vi "Resource Editor.vi"(7 "Load from Initial Path (F)":bool, 10 "Initial Resources":T1[](array[typedef]), 11 "Path":path) -> (2 "Final Resources":T1[](array[typedef]))   [LabVIEW 2026, in "VILab.lvlib"]
doc: "Edits several types of LabVIEW files at a low level, including VI's.\n\nCan also be used as a dialog subVI for editing resource clusters."
uses:
  VILab.lvlib
  CTLs/Resource.ctl
  CTLs/Resource Editor State Data.ctl
  <userlib>/_MGI/Application Control/MGI Gray if/MGI Gray if False.vi
  <vilib>/Utility/error.llb/Three Button Dialog (string).vi
  <vilib>/ErrorRing/Error Ring.xnode
  SubVIs/FaKI State Machine/FaKI State Machine.lvlib
panel:
  in  "Delete":bool
  in  "Add":bool
  in  "Name":string
  in  "Type":string
  in  "ID":i32
  in  "Export":bool
  in  "Import":bool
  in  "Paste":bool
  in  "Copy":bool
  in  "XML":bool
  in  "Fix MD5":bool
  in  "File type":string
  in  "Data":string
  in  "Hex view":bool
  in  "Save":bool
  in  "Load":bool
  in  "Resources":i32(listbox)=-1
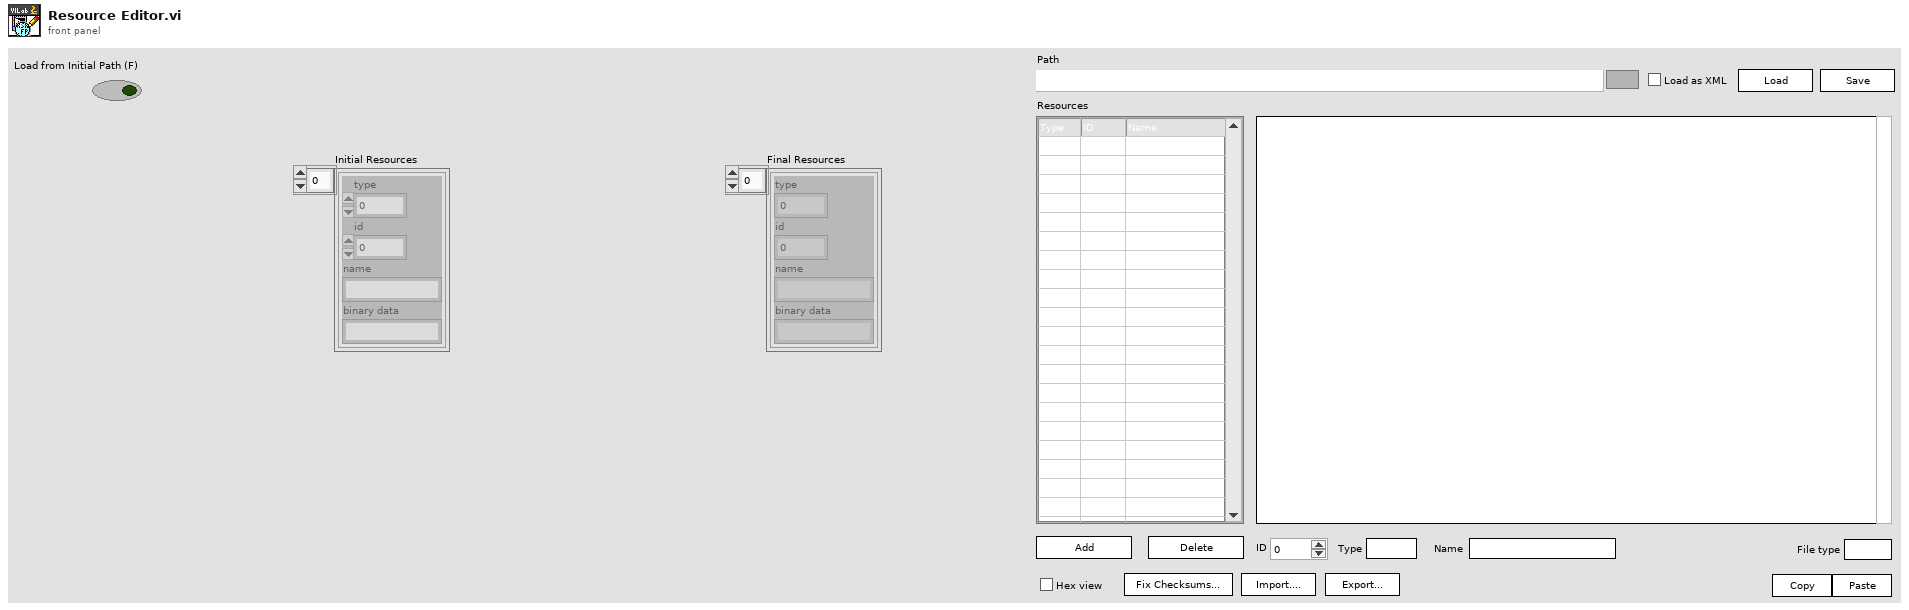
[diagram p1: front panel]
types:
  T1 = typedef "VILab.lvlib/Resource.ctl" = cluster{"type":u32, "id":i32, "name":string, "binary data":string}
  T2 = typedef "VILab.lvlib/Resource Editor State Data.ctl" = cluster{"Core":cluster{"Current VI Reference":refnum<vi>, "Close Panel on Exit?":bool}, "Path":path, "File Type":string, "Active Index":i32, "Active Resource":T1, "All Resources":T1[]}
  T3 = cluster{"format string":string, "Variant":variant}
  T4 = enum32{"Invalid", "Standard", "Closed", "Hidden", "Minimized", "Maximized"}
  T5 = enum32{"invalid app kind", "Development System", "Run Time System", "Student Edition", "Embedded LabVIEW", "Evaluation", "Custom"}
  T6 = enum16{"open", "replace", "create", "open or create", "replace or create", "replace or create with confirmation"}
  T7 = enum16{"Left Button", "Center Button", "Right Button", "Window Close"}
  T8 = enum8{"Enabled", "Disabled", "Disabled and Grayed Out"}
  T9 = typedef "VILab.lvlib/Terminal Counts.ctl" = cluster{"Numbers":u32, "Strings":u32, "Paths":u32}
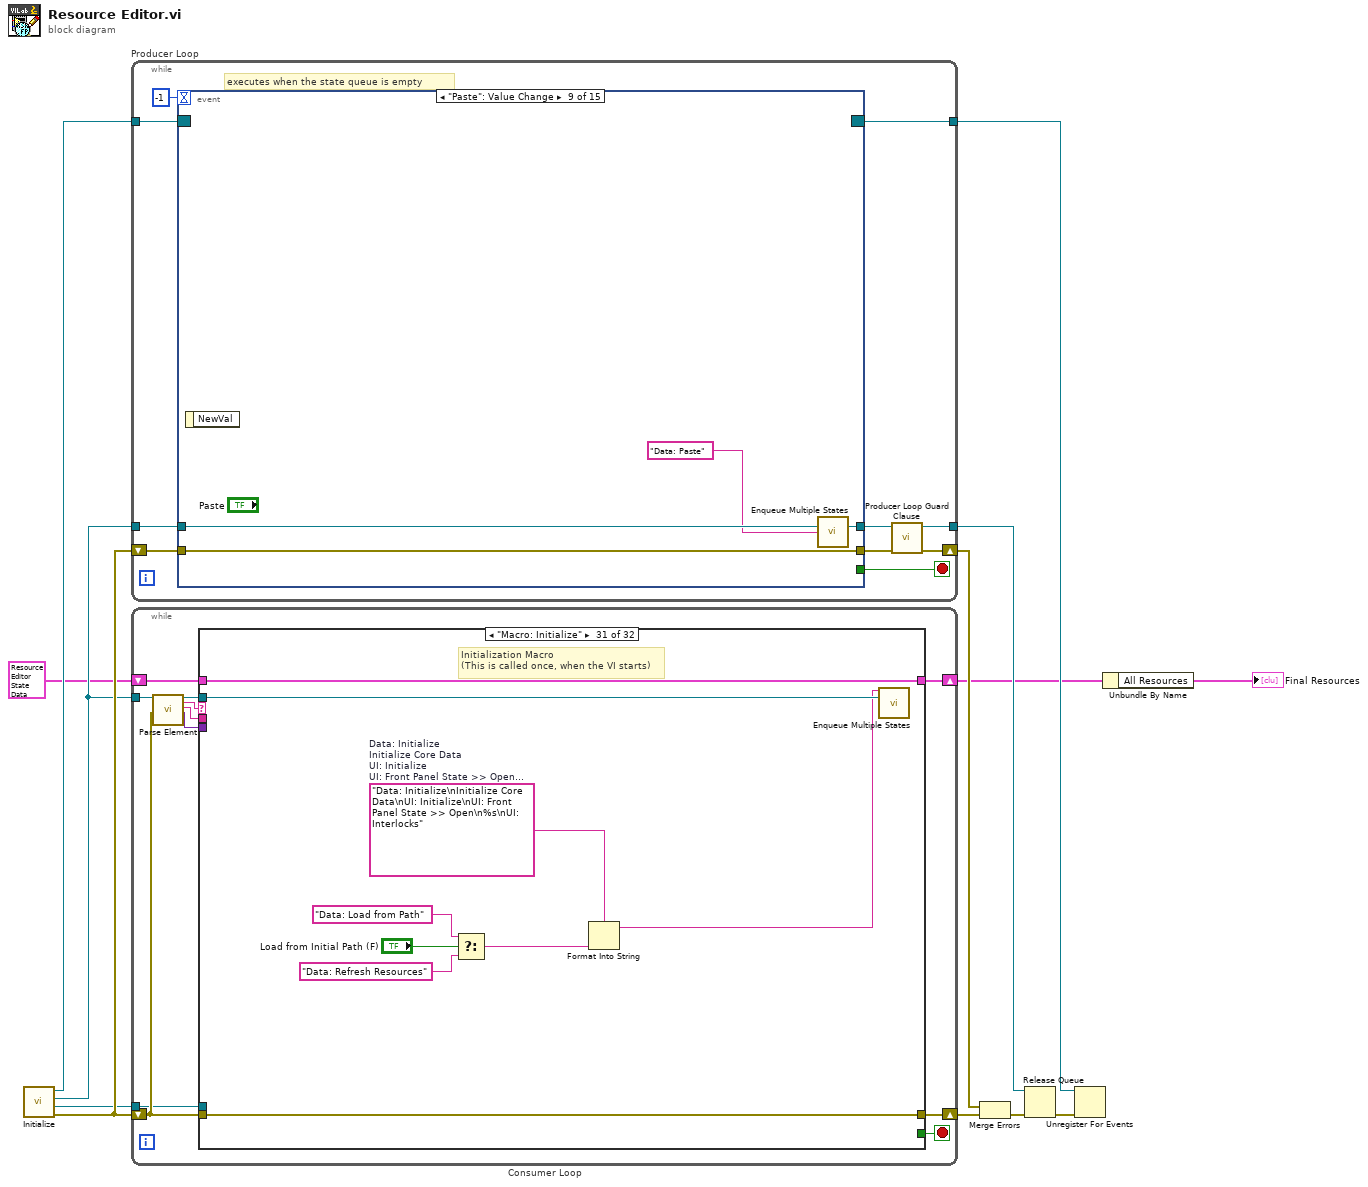
[diagram p0: block diagram]
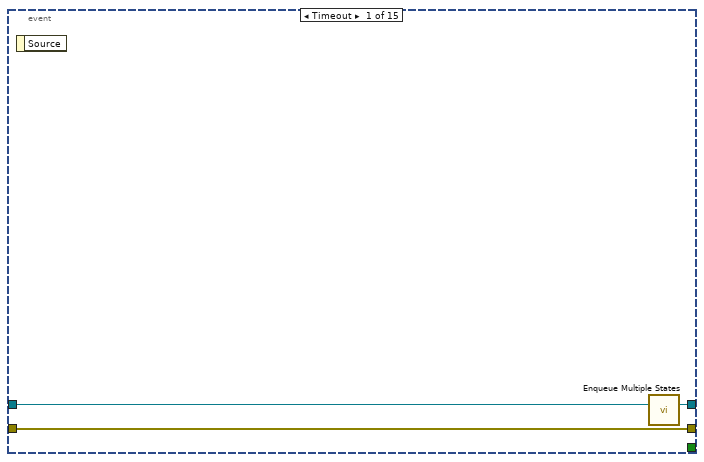
[diagram p2: hidden frame]
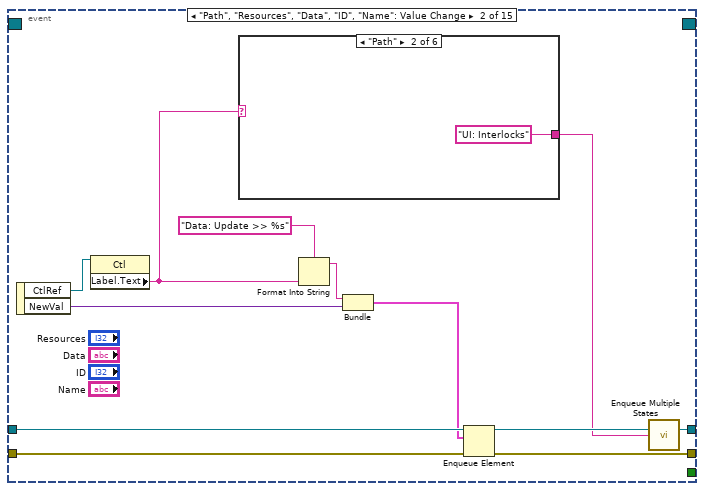
[diagram p3: hidden frame]
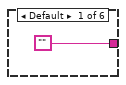
[diagram p4: hidden frame]
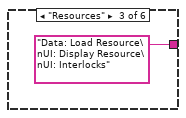
[diagram p5: hidden frame]
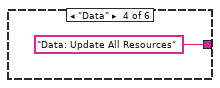
[diagram p6: hidden frame]
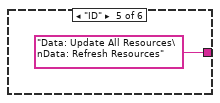
[diagram p7: hidden frame]
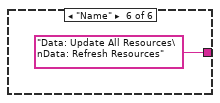
[diagram p8: hidden frame]
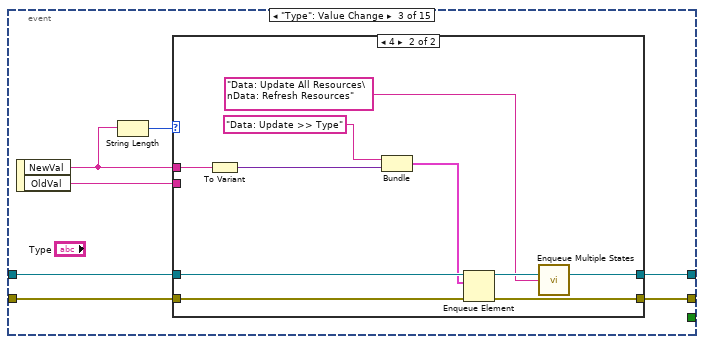
[diagram p9: hidden frame]
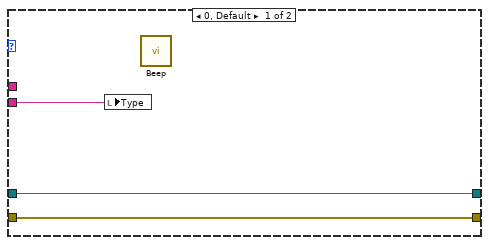
[diagram p10: hidden frame]
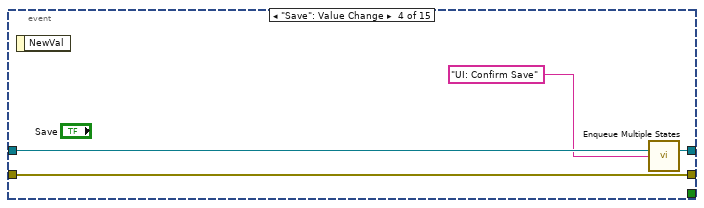
[diagram p11: hidden frame]
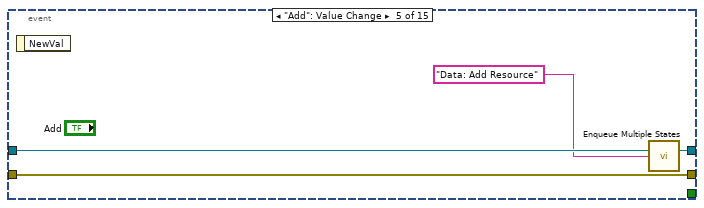
[diagram p12: hidden frame]
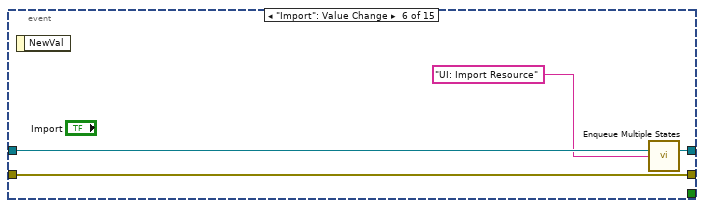
[diagram p13: hidden frame]
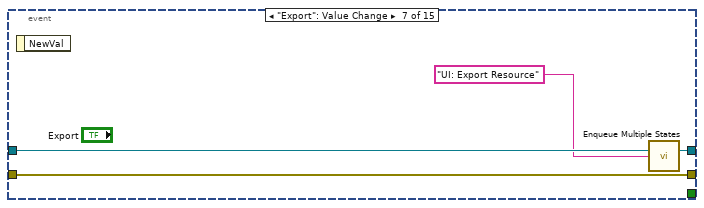
[diagram p14: hidden frame]
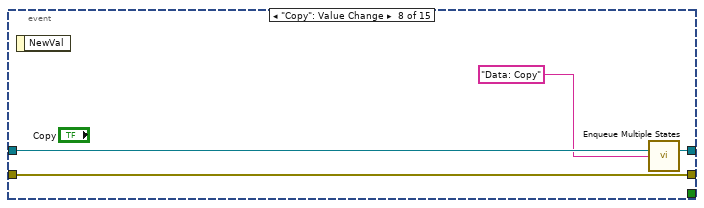
[diagram p15: hidden frame]
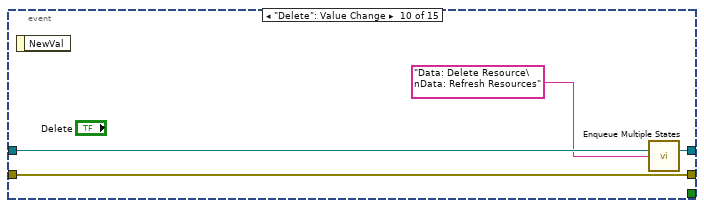
[diagram p16: hidden frame]
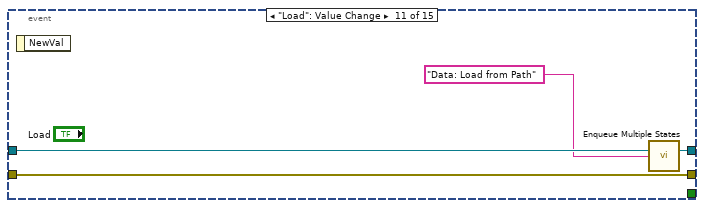
[diagram p17: hidden frame]
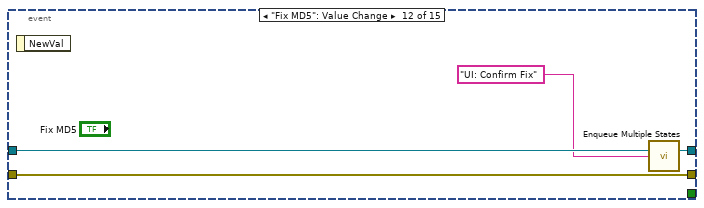
[diagram p18: hidden frame]
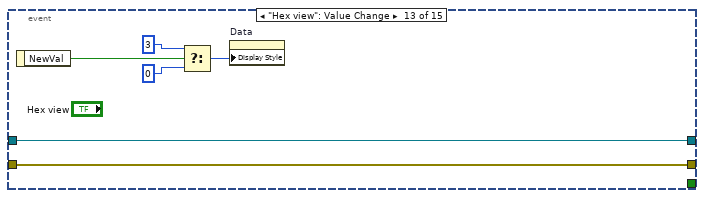
[diagram p19: hidden frame]
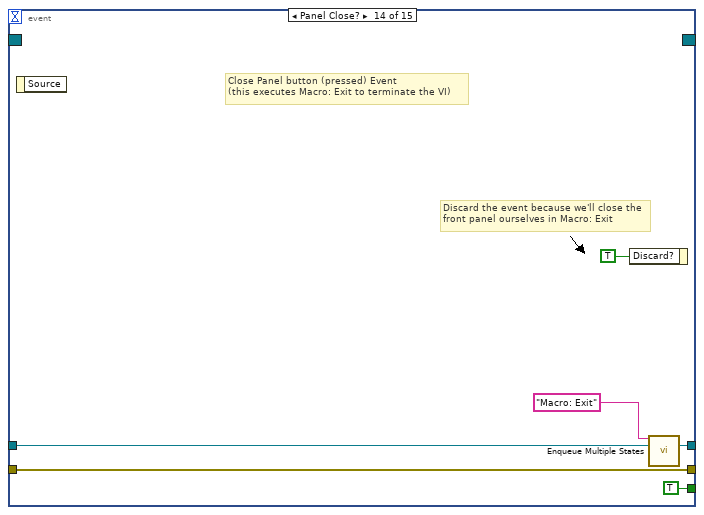
[diagram p20: hidden frame]
diagram:
  n1 = call "Initialize.vi"() -> ("error out"=w9:errorcluster, "Exit Event out"=w6:refnum<user-event>, "queue out"=w8:refnum<queue>, "Event Registration Refnum out"=w7:refnum<event-registration>)  [unwired: 8 in]
  n2 = while "Producer Loop" {
    shift-right: [w18] -> w12
    shift-left: w9 -> [w23]
    tunnel: w7 -> [w15]
    tunnel: w8 -> [w21]
    tunnel: [w16] -> w10
    tunnel: [w14] -> w4
    stop <- w20 stop-if-true
    # "executes when the state queue is empty"
    n3 = event shown="[8] \"Paste\": Value Change" {
      selector: w15 -> [_ _ _ _ _ _ _ _ _ _ _ _ _ _ _]
      dyn-events: [_ _ _ _ _ _ _ _ _ _ _ _ _ _ _] -> w14
      timeout: -1 ("Timeout") -> [_ _ _ _ _ _ _ _ _ _ _ _ _ _ _]
      tunnel: [w24 w36 w49 w67 w71 w75 w79 w83 w87 w91 w95 w99 w106 w112 w117] -> w19
      tunnel: w23 -> [w24 w37 w50 w67 w71 w75 w79 w83 w87 w91 w95 w99 w106 w112 w117]
      tunnel: w21 -> [w25 w35 w48 w66 w70 w74 w78 w82 w86 w90 w94 w98 w105 w109 w115]
      tunnel: [w26 w38 w51 w68 w72 w76 w80 w84 w88 w92 w96 w100 w105 w108 w114] -> w17
      tunnel: [_ _ _ _ _ _ _ _ _ _ _ _ _ TRUE TRUE] -> w20
      event Timeout {
        n4 = event-data() -> ()  [unwired: 1 in, 1 out]
        n5 = call "Enqueue Multiple States.vi"("queue in"=w25) -> ("queue out"=w26:refnum<queue>)  [unwired: 14 in]
      }
      event "Path", "Resources", "Data", "ID", "Name": Value Change {
        n6 = event-data() -> ("CtlRef"=w33:refnum<vi>, "NewVal"=w32:variant)  [unwired: 1 in]
        n7 = property class="Ctl"(reference=w33) -> ("Label.Text"=w29:string)  [unwired: 1 in, 2 out]
        n8 = case shown="\"Path\"" w29 {
          tunnel: ["" "UI: Interlocks" "Data: Load Resource\nUI: Display Resource\nUI: Interlocks" "Data: Update All Resources" "Data: Update All Resources\nData: Refresh Resources" "Data: Update All Resources\nData: Refresh Resources"] -> w27
          frame Default {
          }
          frame "Path" {
          }
          frame "Resources" {
          }
          frame "Data" {
          }
          frame "ID" {
          }
          frame "Name" {
          }
        }
        n9 = Format Into String(format string="Data: Update >> %s", w29) -> (resulting string=w30:string)  [unwired: 2 in, 1 out]
        n10 = Bundle(w30, "NewVal"=w32) -> (w28:cluster{string, "NewVal":variant})  [unwired: 1 in]
        n11 = Enqueue Element(queue=w35, element=w28, error in (no error)=w37) -> (queue out=w34:refnum<queue>, error out=w36:errorcluster)  [unwired: 1 in, 1 out]
        n12 = call "Enqueue Multiple States.vi"("queue in"=w34, "State(s) at Back"=w27) -> ("queue out"=w38:refnum<queue>)  [unwired: 13 in]
      }
      event "Type": Value Change {
        n13 = event-data() -> ("NewVal"=w47:string, "OldVal"=w45:string)  [unwired: 1 in]
        n14 = String Length(string=w47) -> (length=w46:i32)
        n15 = case shown="4" w46 {
          tunnel: [w54 w64] -> w51
          tunnel: w50 -> [w53 w63]
          tunnel: [w53 w62] -> w49
          tunnel: w48 -> [w54 w61]
          tunnel: w47 -> [_ w56]
          tunnel: w45 -> [w52 _]
          frame 0, Default {
            n16 = local write "Type"(w52) -> ()
            n17 = call <vilib>:"Beep.vi"() -> ()  [unwired: 12 in]
          }
          frame 4 {
            n18 = To Variant(anything=w56) -> (Variant=w55:variant)
            n19 = Bundle("format string"="Data: Update >> Type", "Variant"=w55) -> (w58:T3)  [unwired: 1 in]
            n20 = Enqueue Element(queue=w61, element=w58, error in (no error)=w63) -> (queue out=w60:refnum<queue>, error out=w62:errorcluster)  [unwired: 1 in, 1 out]
            n21 = call "Enqueue Multiple States.vi"("queue in"=w60, "State(s) at Back"="Data: Update All Resources\nData: Refresh Resources") -> ("queue out"=w64:refnum<queue>)  [unwired: 13 in]
          }
        }
      }
      event "Save": Value Change {
        n22 = event-data() -> ()  [unwired: 1 in, 1 out]
        n23 = call "Enqueue Multiple States.vi"("queue in"=w66, "State(s) at Back"="UI: Confirm Save") -> ("queue out"=w68:refnum<queue>)  [unwired: 13 in]
      }
      event "Add": Value Change {
        n24 = event-data() -> ()  [unwired: 1 in, 1 out]
        n25 = call "Enqueue Multiple States.vi"("queue in"=w70, "State(s) at Back"="Data: Add Resource") -> ("queue out"=w72:refnum<queue>)  [unwired: 13 in]
      }
      event "Import": Value Change {
        n26 = event-data() -> ()  [unwired: 1 in, 1 out]
        n27 = call "Enqueue Multiple States.vi"("queue in"=w74, "State(s) at Back"="UI: Import Resource") -> ("queue out"=w76:refnum<queue>)  [unwired: 13 in]
      }
      event "Export": Value Change {
        n28 = event-data() -> ()  [unwired: 1 in, 1 out]
        n29 = call "Enqueue Multiple States.vi"("queue in"=w78, "State(s) at Back"="UI: Export Resource") -> ("queue out"=w80:refnum<queue>)  [unwired: 13 in]
      }
      event "Copy": Value Change {
        n30 = event-data() -> ()  [unwired: 1 in, 1 out]
        n31 = call "Enqueue Multiple States.vi"("queue in"=w82, "State(s) at Back"="Data: Copy") -> ("queue out"=w84:refnum<queue>)  [unwired: 13 in]
      }
      event "Paste": Value Change {
        n32 = event-data() -> ()  [unwired: 1 in, 1 out]
        n33 = call "Enqueue Multiple States.vi"("queue in"=w86, "State(s) at Back"="Data: Paste") -> ("queue out"=w88:refnum<queue>)  [unwired: 13 in]
      }
      event "Delete": Value Change {
        n34 = event-data() -> ()  [unwired: 1 in, 1 out]
        n35 = call "Enqueue Multiple States.vi"("queue in"=w90, "State(s) at Back"="Data: Delete Resource\nData: Refresh Resources") -> ("queue out"=w92:refnum<queue>)  [unwired: 13 in]
      }
      event "Load": Value Change {
        n36 = event-data() -> ()  [unwired: 1 in, 1 out]
        n37 = call "Enqueue Multiple States.vi"("queue in"=w94, "State(s) at Back"="Data: Load from Path") -> ("queue out"=w96:refnum<queue>)  [unwired: 13 in]
      }
      event "Fix MD5": Value Change {
        n38 = event-data() -> ()  [unwired: 1 in, 1 out]
        n39 = call "Enqueue Multiple States.vi"("queue in"=w98, "State(s) at Back"="UI: Confirm Fix") -> ("queue out"=w100:refnum<queue>)  [unwired: 13 in]
      }
      event "Hex view": Value Change {
        n40 = event-data() -> ("NewVal"=w101:bool)  [unwired: 1 in]
        n41 = Select(t=u32 3 ("Display Style"), s=w101, f=u32 0 ("Display Style")) -> (s? t:f=w104:u32)
        n42 = property on="Data" class="Str"("Display Style"=w104) -> ()  [unwired: 2 in, 2 out]
      }
      event Panel Close? {
        # "Discard the event because we'll close the front panel ourselves in Macro: Exit"
        # "Close Panel button (pressed) Event\n(this executes Macro: Exit to terminate the VI)"
        n43 = event-data() -> ()  [unwired: 1 in, 1 out]
        n44 = event-data("Discard?"=TRUE) -> ()  [unwired: 1 in, 1 out]
        n45 = call "Enqueue Multiple States.vi"("State(s) at Front"="Macro: Exit", "queue in"=w109) -> ("queue out"=w108:refnum<queue>)  [unwired: 13 in]
      }
      event User Event {
        # "\"Exit\" Dynamic Event registered\n(this executes Macro: Exit to terminate the VI)"
        n46 = event-data() -> ()  [unwired: 1 in, 5 out]
        n47 = call "Enqueue Multiple States.vi"("State(s) at Front"="Macro: Exit", "queue in"=w115) -> ("queue out"=w114:refnum<queue>)  [unwired: 13 in]
      }
    }
    n48 = call "Producer Loop Guard Clause.vi"("error in (no error)"=w19, "queue in"=w17) -> ("error out"=w18:errorcluster, "queue out"=w16:refnum<queue>)  [unwired: 8 in]
  }
  n49 = while "Consumer Loop" {
    shift-right: [w125] -> w2
    shift-left: T2 {"Core"={"Current VI Reference"=refnum, "Close Panel on Exit?"=FALSE}, "Path"=path "", "File Type"="", "Active Index"=0, "Active Resource"={"type"=0, "id"=0, "name"="", "binary data"=""}, "All Resources"=[]} ("Resource Editor State Data") -> [w124]
    shift-right: [w128] -> w13
    shift-left: w9 -> [w127]
    tunnel: w8 -> [w123]
    tunnel: w6 -> [w118]
    stop <- w126 stop-if-true
    n50 = call "Parse Element.vi"("queue in"=w123, "error in (no error)"=w127) -> ("queue out"=w122:refnum<queue>, "State"=w121:string, "Arg"=w120:string, "Data"=w119:variant)  [unwired: 14 in]
    n51 = case shown="\"Macro: Initialize\"" w121 {
      selector: w121 -> [_ w133 _ _ _ _ _ _ _ _ _ _ _ _ _ _ _ _ _ _ _ _ _ _ _ _ _ _ _ _ _ _]
      tunnel: w122 -> [w129 w132 w142 w158 _ w164 _ _ w243 _ _ _ _ _ w297 w327 _ _ _ _ w415 w419 w428 w431 w440 _ _ _ _ w586 w595 w602]
      tunnel: w120 -> [_ _ _ w154 _ _ _ w175 _ _ _ _ _ _ _ _ _ _ _ _ _ _ _ w432 w441 _ _ _ _ _ _ _]
      tunnel: w124 -> [w130 w135 w148 w159 w162 w165 w169 w176 w242 w255 w266 w272 w282 w288 w304 w330 w344 w355 w364 w396 w416 w420 w429 w433 w443 w518 w523 w535 w551 w587 w596 w606]
      tunnel: [w131 w140 w153 errorcluster {"status"=FALSE, "code"=0, "source"=""} ("error out") w163 w166 w170 w171 w232 w257 w267 w273 w283 w289 w298 w328 w342 w356 w365 w390 w418 w421 w430 w434 w444 w516 w529 w530 w552 w588 w597 w607] -> w128
      tunnel: w127 -> [w131 w139 w153 w157 w163 w166 w170 w174 w234 w257 w267 w273 w283 w289 w299 w329 w345 w356 w365 w397 w414 w421 w430 w435 w445 w522 w529 w532 w552 w588 w597 w607]
      tunnel: [_ _ _ _ TRUE _ _ _ _ _ _ _ _ _ _ _ _ _ _ _ _ _ _ _ _ _ _ _ _ _ _ _] -> w126
      tunnel: [w130 w135 w152 w159 w162 w165 w168 w172 w238 w255 w265 w271 w281 w287 w304 w330 w343 w354 w363 w395 w416 w420 w429 w433 w443 w518 w523 w535 w550 w587 w596 w606] -> w125
      tunnel: w119 -> [_ _ _ w155 _ _ _ w173 _ _ _ _ _ _ _ _ w341 _ _ w394 _ _ _ _ _ _ _ _ _ _ _ _]
      tunnel: w118 -> [_ _ _ _ _ _ _ _ _ _ _ _ _ _ _ _ _ _ _ _ w413 _ _ _ _ _ _ _ _ _ _ _]
      frame "---------- Core ----------" {
        # "Do not put any code in this frame.\n(it is a separator no-op)"
        n52 = call "Enqueue Multiple States.vi"("queue in"=w129) -> ()  [unwired: 14 in, 1 out]
      }
      frame Default {
        w137 = 42 items=["No error", "Argument error", "Memory is full", "Out of zone", "End of file", "File already open", "Generic file I/O error", "File not found", "File permission error", "Disk is full", "Duplicate path", "Too many files open", "System feature not enabled", "Resource file not found", "Cannot add resource", "Resource not found", "Image not found", "Image memory error", "Pen does not exist", "Config type invalid", "Config token not found", "Config parse error", "Config memory error", "Bad external code format", "Bad external code offset", "External code not present", "Null window", "Destroy window error", "Null menu", "Print aborted", "Bad print record", "Print driver error", "Windows error during printing", "Memory error during printing", "Print dialog error", "Generic print error", "Invalid device refnum", "Device not found", "Device parameter error", "Device unit error", "Cannot open device", "Device call aborted", "Generic error", "Cancelled by user", "Object ID too low", "Object ID too high", "Object not in heap", "Unknown heap", "Unknown object (invalid DefProc)", "Unknown object (DefProc not in table)", "Message out of range", "Invalid (null) method", "Unknown message", "Manager call not supported", "Bad address", "Network operation in progress", "Network operation timed out", "Connection is busy", "Network attribute not supported", "Network error", "Address in use", "System out of memory", "Connection aborted", "Connection refused", "Not connected", "Already connected", "Connection closed", "Initialization error (interapplication manager)", "Bad occurrence", "Wait on unbound occurrence handler", "Occurrence queue overflow", "Datalog type conflict", "Unused", "Unrecognized type (interapplication manager)", "Memory corrupt", "Failed to make temporary DLL", "Old CIN version", "Drag socket not found", "Failed to load drop-object", "Failed to register OLE object", "Failed to release OLE object", "Format specifier type mismatch", "Unknown format specifier", "Too few format specifiers", "Too many format specifiers", "Scan failed", "Newer CIN version", "Error converting to variant", "Runtime menu error", "Password tampered", "Variant attribute not found", "Incompatible variant data type", "Event data is not available", "Event Store is not present", "Occurrence is not found", "Event Queue is not created", "Event info is not available", "Refnum passed is NULL", "Error retrieving Class GUID", "Error retrieving CoClass GUID", "Error retrieving TypeLib GUID.", "Bad built application magic bytes.", "Specific driver is different from the specific driver associated with the Logical Name.", "There is no session opened to the class driver.", "Max Error", "MAX - Error with config objects", "MAX - Error loading configuration", "MAX - Group not supported"]
        # "Current State"
        # "Do not delete, rename, or modify this frame.\n(this is used to capture unhandled states and typos)"
        # "Handle mistyped state name (developer tool)"
        n53 = Format Into String(format string="Software Exception: Unhandled State \"%s\"." ("message"), error in=w139, w133) -> (resulting string=w136:string, error out=w141:errorcluster)  [unwired: 1 in]
        n54 = call <vilib>:"Error Cluster From Error Code.vi"("show call chain? (False)"=TRUE, "error in (no error)"=w141, "error message (\"\")"=w136, "error code (0)"=w137) -> ("error out"=w140:errorcluster)  [unwired: 5 in]
        n55 = call "Enqueue Multiple States.vi"("queue in"=w132) -> ()  [unwired: 14 in, 1 out]
      }
      frame "Initialize Core Data" {
        # "Do not delete, rename, or modify this frame.\n(this is used to determine panel behavior on exit)"
        # "originally closed?"
        # "exe?"
        # "If panel starts closed or is an EXE, then close it when we exit"
        n56 = property class="VI"() -> ("FP.State"=w145:T4)  [unwired: 2 in, 2 out]
        n57 = property class="App"() -> ("App.Kind"=w151:T5)  [unwired: 2 in, 2 out]
        n58 = control-ref of="Current VI Reference"() -> (w146:refnum<vi>)
        n59 = Equal?(x=w145, y=T4."Closed" ("Front Panel Window:State")) -> (x = y?=w143:bool)
        n60 = Equal?(x=w151, y=T5."Run Time System" ("Application:Kind")) -> (x = y?=w149:bool)
        n61 = Or(x=w143, y=w149) -> (x .or. y?=w147:bool)
        n62 = Bundle By Name(cluster=w148, "Core.Current VI Reference"=w146, "Core.Close Panel on Exit?"=w147) -> (w152:T2)
        n63 = call "Enqueue Multiple States.vi"("queue in"=w142) -> ()  [unwired: 14 in, 1 out]
      }
      frame "Error Handler" {
        # "Unhandled Error -- Display it"
        # "Handle any errors here.\nYou can also output any states to clean-up after errors occur"
        # "Clear error"
        n64 = call "Build Error Message.vi"("error in (no error)"=w157, "Data"=w155, "Arg"=w154) -> ("error out"=w156:errorcluster)  [unwired: 8 in]
        n65 = call <vilib>:"General Error Handler.vi"("error in (no error)"=w156) -> ()  [unwired: 10 in, 5 out]
        n66 = call "Enqueue Multiple States.vi"("queue in"=w158) -> ()  [unwired: 14 in, 1 out]
      }
      frame "Exit" {
        # "Do not put any code in this frame.\n(No errors that occur here will be handled.)"
      }
      frame "---------- Data ----------" {
        # "Do not put any code in this frame.\n(It is a separator no-op. You can make a copy of this frame to create a new Data frame)"
        n67 = call "Enqueue Multiple States.vi"("queue in"=w164) -> ()  [unwired: 14 in, 1 out]
      }
      frame "Data: Initialize" {
        # "Initialize the shift-register data, here."
        n68 = Bundle By Name(cluster=w169, "All Resources"="Initial Resources") -> (w168:T2)
      }
      frame "Data: Update" {
        n69 = case shown="\"Name\"" w175 {
          selector: w175 -> [w177 _ _ _ _ _ _]
          tunnel: w176 -> [w179 w190 w197 w204 w213 w220 w227]
          tunnel: w174 -> [_ w193 w200 w207 w216 w223 w230]
          tunnel: w173 -> [_ w191 w198 w205 w214 w221 w228]
          tunnel: [w179 w189 w196 w203 w212 w219 w226] -> w172
          tunnel: [w178 w187 w194 w201 w211 w218 w225] -> w171
          frame Default {
            n70 = xnode "Error Ring"("parameter 0"=w177) -> ("error out"=w178:errorcluster)
          }
          frame "Path" {
            n71 = Variant To Data(error in=w193, type=path "", Variant=w191) -> (data=w188:path, error out=w187:errorcluster)
            n72 = Bundle By Name(cluster=w190, "Path"=w188) -> (w189:T2)
          }
          frame "Resources" {
            n73 = Variant To Data(error in=w200, type=0, Variant=w198) -> (data=w195:i32, error out=w194:errorcluster)
            n74 = Bundle By Name(cluster=w197, "Active Index"=w195) -> (w196:T2)
          }
          frame "Data" {
            n75 = Variant To Data(error in=w207, type="", Variant=w205) -> (data=w202:string, error out=w201:errorcluster)
            n76 = Bundle By Name(cluster=w204, "Active Resource.binary data"=w202) -> (w203:T2)
          }
          frame "Type" {
            n77 = Variant To Data(error in=w216, type="", Variant=w214) -> (data=w209:string, error out=w211:errorcluster)
            n78 = Type Cast(type=u32 0, x=w209) -> (*(type *) &x=w208:u32)
            n79 = Bundle By Name(cluster=w213, "Active Resource.type"=w208) -> (w212:T2)
          }
          frame "ID" {
            n80 = Variant To Data(error in=w223, type=0, Variant=w221) -> (data=w217:i32, error out=w218:errorcluster)
            n81 = Bundle By Name(cluster=w220, "Active Resource.id"=w217) -> (w219:T2)
          }
          frame "Name" {
            n82 = Variant To Data(error in=w230, type="", Variant=w228) -> (data=w224:string, error out=w225:errorcluster)
            n83 = Bundle By Name(cluster=w227, "Active Resource.name"=w224) -> (w226:T2)
          }
        }
      }
      frame "Data: Load from Path" {
        n84 = case shown="True" "XML" {
          tunnel: "Path" -> [w245 w253]
          tunnel: [w245 w248] -> w239
          tunnel: w234 -> [w244 w247]
          tunnel: [w244 w246] -> w233
          frame False {
          }
          frame True {
            n85 = Open VI Reference(vi path=w253, error in (no error)=w247) -> (vi reference=w252:refnum<vi>, error out=w251:errorcluster)  [unwired: 4 in]
            n86 = call "Save VI with XML Heaps.vi"("error in (no error)"=w251, "VI Refnum In"=w252) -> ("error out"=w250:errorcluster, "VI Path out"=w248:path, "VI Refnum Out"=w249:refnum<vi>)  [unwired: 7 in]
            n87 = Close Reference(reference=w249, error in (no error)=w250) -> (error out=w246:errorcluster)
          }
        }
        n88 = property on="Resources" class="MCListbox (strict)"("Val(Sgnl)"=0 ("Value (Signaling)")) -> ()  [unwired: 2 in, 2 out]
        n89 = call "Load Resource File.vi"("error in (no error)"=w233, "Resource File"=w239) -> ("error out"=w232:errorcluster, "File Type"=w231:string, "Resources"=w237:T1[])  [unwired: 7 in]
        n90 = Bundle By Name(cluster=w242, "All Resources"=w237, "File Type"=w231) -> (w238:T2)
        n91 = local write "File type"(w231) -> ()
        n92 = call "Enqueue Multiple States.vi"("queue in"=w243, "State(s) at Back"="Data: Refresh Resources") -> ()  [unwired: 13 in, 1 out]
      }
      frame "Data: Refresh Resources" {
        n93 = Unbundle By Name(w255) -> ("All Resources"=w254:T1[])
        n94 = for {
          tunnel: [w264] -> w256 mode=indexing
          tunnel: w254 -> [w260] mode=indexing
          n95 = Unbundle By Name(w260) -> ("type"=w263:u32, "id"=w259:i32, "name"=w258:string)
          n96 = Type Cast(x=w263) -> (*(type *) &x=w261:string)  [unwired: 1 in]
          n97 = Number To Decimal String(number=w259) -> (decimal integer string=w262:string)  [unwired: 1 in]
          n98 = Build Array(w261, w262, w258) -> (w264:string[])
        }
        n99 = property on="Resources" class="MCListbox (strict)"("ItemNames"=w256) -> ()  [unwired: 2 in, 2 out]
      }
      frame "Data: Delete Resource" {
        n100 = in-place {
          n101 = in-place-cluster #1(w266) -> ("All Resources"=w270:T1[], "Active Index"=w268:i32)
          n102 = Delete From Array(array=w270, index=w268) -> (array with subset deleted=w269:T1[])  [unwired: 1 in, 1 out]
          n103 = in-place-cluster #1("All Resources"=w269, "Active Index"=w268) -> (w265:T2)
        }
      }
      frame "Data: Add Resource" {
        n104 = in-place {
          n105 = in-place-cluster #2(w272) -> ("All Resources"=w276:T1[], "Active Index"=w274:i32)
          n106 = property on="Resources" class="MCListbox (strict)"() -> ("ItemNames"=w280:string[][])  [unwired: 2 in, 2 out]
          n107 = Insert Into Array(array=w280, index (row)=w274, new element=string[] ["NewR", "0", ""]) -> (w279:string[][])  [unwired: 1 in]
          n108 = Insert Into Array(array=w276, index=w274, new element=T1 {"type"=1315272530, "id"=0, "name"="", "binary data"=""} ("element")) -> (w275:T1[])
          n109 = property on="Resources" class="MCListbox (strict)"("ItemNames"=w279, "Val(Sgnl)"=w274) -> ()  [unwired: 2 in, 2 out]
          n110 = in-place-cluster #2("All Resources"=w275, "Active Index"=w274) -> (w271:T2)
        }
      }
      frame "Data: Load Resource" {
        n111 = in-place {
          n112 = in-place-cluster #3(w282) -> ("All Resources"=w285:T1[], "Active Index"=w286:i32)  [unwired: 1 out]
          n113 = Index Array(array=w285, index=w286) -> (element=w284:T1)
          n114 = in-place-cluster #3("Active Resource"=w284, "All Resources"=w285, "Active Index"=w286) -> (w281:T2)
        }
      }
      frame "Data: Update All Resources" {
        n115 = in-place {
          n116 = in-place-cluster #4(w288) -> ("Active Resource"=w292:T1, "All Resources"=w295:T1[], "Active Index"=w294:i32)
          n117 = in-place {
            in-place-border: w292 -> [w296]
            in-place-border: [w296] -> w290
            n118 = in-place-array #5(w295, w294) -> ()  [unwired: 1 out]
            n119 = in-place-array #5(w296) -> (w291:T1[], w293:i32)
          }
          n120 = in-place-cluster #4("Active Resource"=w290, "All Resources"=w291, "Active Index"=w293) -> (w287:T2)
        }
      }
      frame "UI: Import Resource" {
        n121 = call "Select File for Import"("button label"="Open") -> ("selected path"=w302:path, "cancelled"=w303:bool, "error out"=w301:errorcluster)  [unwired: 11 in, 1 out]
        n122 = call <vilib>:"Clear Errors.vi"("error in (no error)"=w301) -> ()  [unwired: 5 in, 2 out]
        n123 = case shown="False" w303 {
          tunnel: w302 -> [w314 _]
          tunnel: w299 -> [w311 w322]
          tunnel: [w310 w322] -> w298
          tunnel: w297 -> [w309 _]
          frame False {
            n124 = Open/Create/Replace File(file path (use dialog)=w314, error in=w311, access (0:read/write)=enum16{"read/write", "read-only", "write-only"}."read-only") -> (refnum out=w321:refnum<file>, error out=w320:errorcluster)  [unwired: 3 in, 1 out]
            n125 = Read from Binary File(5:u8 0, 8:w320, 10:-1 ("count (1)"), 11:w321) -> (0:w318:errorcluster, 2:w313:u8[], 3:w319:refnum<file>)  [unwired: 2 in, 1 out]
            n126 = Byte Array To String(unsigned byte array=w313) -> (string=w307:string)
            n127 = To Variant(anything=w307) -> (Variant=w305:variant)
            n128 = Close File(refnum=w319, error in=w318) -> (error out=w312:errorcluster)  [unwired: 1 out]
            n129 = Bundle("Data: Import Resource", "Variant"=w305) -> (w306:cluster{string, "Variant":variant})  [unwired: 1 in]
            n130 = Enqueue Element(queue=w309, element=w306, error in (no error)=w312) -> (error out=w310:errorcluster)  [unwired: 1 in, 2 out]
          }
          frame True {
          }
        }
      }
      frame "UI: Export Resource" {
        n131 = call "Select File for Export"("button label"="Save") -> ("selected path"=w324:path, "cancelled"=w323:bool, "error out"=w326:errorcluster)  [unwired: 11 in, 1 out]
        n132 = call <vilib>:"Clear Errors.vi"("error in (no error)"=w326) -> ()  [unwired: 5 in, 2 out]
        n133 = case shown="False" w323 {
          tunnel: w324 -> [w331 _]
          tunnel: w329 -> [w332 w338]
          tunnel: [w337 w338] -> w328
          tunnel: w327 -> [w336 _]
          frame False {
            n134 = To Variant(anything=w331) -> (Variant=w333:variant)
            n135 = Bundle("Data: Export Resource", "Variant"=w333) -> (w334:cluster{string, "Variant":variant})  [unwired: 1 in]
            n136 = Enqueue Element(queue=w336, element=w334, error in (no error)=w332) -> (error out=w337:errorcluster)  [unwired: 1 in, 2 out]
          }
          frame True {
          }
        }
      }
      frame "Data: Import Resource" {
        n137 = Variant To Data(error in=w345, type="", Variant=w341) -> (data=w339:string, error out=w342:errorcluster)
        n138 = in-place {
          in-place-border: w339 -> [w346]
          n139 = in-place-cluster #6(w344) -> ("All Resources"=w350:T1[], "Active Index"=w349:i32)
          n140 = in-place {
            in-place-border: w346 -> [w351]
            n141 = in-place-array #7(w350, w349) -> (w353:T1)
            n142 = Bundle By Name(cluster=w353, "binary data"=w351) -> (w352:T1)
            n143 = local write "Data"(w351) -> ()
            n144 = in-place-array #7(w352) -> (w348:T1[], w347:i32)
          }
          n145 = in-place-cluster #6("All Resources"=w348, "Active Index"=w347) -> (w343:T2)
        }
      }
      frame "Data: Copy" {
        n146 = in-place {
          n147 = in-place-cluster #8(w355) -> ("All Resources"=w361:T1[], "Active Index"=w362:i32)
          n148 = Index Array(array=w361, index=w362) -> (element=w358:T1)
          n149 = Unbundle By Name(w358) -> ("binary data"=w357:string)
          n150 = String Subset(string=w357, offset (0)=4) -> (substring=w360:string)  [unwired: 1 in]
          n151 = invoke class="App" method="Clipboard.Write"("Param 0"=w360) -> ()  [unwired: 3 in, 4 out]
          n152 = in-place-cluster #8("All Resources"=w361, "Active Index"=w362) -> (w354:T2)
        }
      }
      frame "Data: Paste" {
        n153 = in-place {
          n154 = in-place-cluster #9(w364) -> ("All Resources"=w369:T1[], "Active Index"=w367:i32)
          n155 = invoke class="App" method="Clipboard.Read"() -> (error out=w376:errorcluster, "Read Clipbrd"=w371:string)  [unwired: 3 in, 1 out]
          n156 = String Length(string=w371) -> (length=w373:i32)
          n157 = Type Cast(x=w373) -> (*(type *) &x=w374:string)  [unwired: 1 in]
          n158 = call "Is Big Endian.vi"() -> ("big endian"=w375:bool)
          n159 = case shown="True" w375 {
            tunnel: w374 -> [w377 w379]
            tunnel: [w377 w378] -> w370
            frame False {
            }
            frame True {
              n160 = Reverse String(1:w379) -> (0:w378:string)
            }
          }
          n161 = Concatenate Strings(w370, w371) -> (w372:string)
          n162 = case shown="No Error" w376 {
            tunnel: w372 -> [w382 _]
            tunnel: w369 -> [w383 w389]
            tunnel: w367 -> [w384 w388]
            tunnel: [w381 w389] -> w368
            tunnel: [w380 w388] -> w366
            frame No Error {
              n163 = in-place {
                in-place-border: w382 -> [w385]
                n164 = in-place-array #10(w383, w384) -> (w386:T1)
                n165 = local write "Data"(w385) -> ()
                n166 = Bundle By Name(cluster=w386, "binary data"=w385) -> (w387:T1)
                n167 = in-place-array #10(w387) -> (w381:T1[], w380:i32)
              }
            }
            frame Error {
            }
          }
          n168 = in-place-cluster #9("All Resources"=w368, "Active Index"=w366) -> (w363:T2)
        }
      }
      frame "Data: Export Resource" {
        n169 = Variant To Data(error in=w397, type=path "", Variant=w394) -> (data=w392:path, error out=w391:errorcluster)
        n170 = in-place {
          in-place-border: w392 -> [w411]
          in-place-border: w391 -> [w400]
          in-place-border: [w399] -> w390
          n171 = in-place-cluster #11(w396) -> ("All Resources"=w402:T1[], "Active Index"=w403:i32)
          n172 = Index Array(array=w402, index=w403) -> (element=w407:T1)
          n173 = Unbundle By Name(w407) -> ("binary data"=w398:string)
          n174 = Open/Create/Replace File(file path (use dialog)=w411, error in=w400, operation (0:open)=T6."replace or create", access (0:read/write)=enum16{"read/write", "read-only", "write-only"}."write-only") -> (refnum out=w406:refnum<file>, error out=w410:errorcluster)  [unwired: 2 in, 1 out]
          n175 = Write to Binary File(file (use dialog)=w406, data=w398, error in=w410, 5:FALSE ("prepend array or string size? (T)")) -> (refnum out=w409:refnum<file>, error out=w408:errorcluster)  [unwired: 2 in, 1 out]
          n176 = Close File(refnum=w409, error in=w408) -> (error out=w399:errorcluster)  [unwired: 1 out]
          n177 = in-place-cluster #11("All Resources"=w402, "Active Index"=w403) -> (w395:T2)
        }
      }
      frame "Data: Cleanup" {
        # "Cleanup any data and references, here.\n(this is called automatically, by the Macro: Exit)"
        n178 = Destroy User Event(user event=w413, error in=w414) -> (error out=w412:errorcluster)
        n179 = Unbundle By Name(w416) -> ("Core.Current VI Reference"=w417:refnum<vi>)
        n180 = Close Reference(reference=w417, error in (no error)=w412) -> (error out=w418:errorcluster)
        n181 = call "Enqueue Multiple States.vi"("queue in"=w415) -> ()  [unwired: 14 in, 1 out]
      }
      frame "---------- UI ----------" {
        # "Do not put any code in this frame.\n(It is a separator no-op. You can make a copy of this frame to create a new UI frame)"
        n182 = call "Enqueue Multiple States.vi"("queue in"=w419) -> ()  [unwired: 14 in, 1 out]
      }
      frame "UI: Initialize" {
        w427 = T8."Disabled and Grayed Out" ("Disabled")
        # "Initialize the User Interface, here.\n(this is called automatically, by the Macro: Init)"
        n183 = local read "Hex view"() -> (w422:bool)
        n184 = property on="Resources" class="MCListbox (strict)"("ItemNames"=string[][] [] ("Item Names")) -> ()  [unwired: 2 in, 2 out]
        n185 = Select(t=u32 3 ("Display Style"), s=w422, f=u32 0 ("Display Style")) -> (s? t:f=w423:u32)
        n186 = property on="Data" class="Str"("Display Style"=w423) -> ()  [unwired: 2 in, 2 out]
        n187 = property on="Copy" class="Bool"("DisabledEnum"=w427) -> ()  [unwired: 2 in, 2 out]
        n188 = property on="Paste" class="Bool"("DisabledEnum"=w427) -> ()  [unwired: 2 in, 2 out]
        n189 = call "Enqueue Multiple States.vi"("queue in"=w428) -> ()  [unwired: 14 in, 1 out]
      }
      frame "UI: Cursor Set" {
        # "Argument"
        # "Set and Unset Cursor Busy.\n(Usage: \"UI: Cursor Set >> Busy|Idle\")"
        n190 = case shown="\"Idle\", Default" w432 {
          tunnel: w435 -> [w437 w439]
          tunnel: [w436 w438] -> w434
          frame "Idle", Default {
            n191 = call <vilib>:"Unset Busy.vi"("error in (no error)"=w437) -> ("error out"=w436:errorcluster)  [unwired: 10 in]
          }
          frame "Busy" {
            n192 = call <vilib>:"Set Busy.vi"("error in (no error)"=w439) -> ("error out"=w438:errorcluster)  [unwired: 9 in, 1 out]
          }
        }
        n193 = call "Enqueue Multiple States.vi"("queue in"=w431) -> ()  [unwired: 14 in, 1 out]
      }
      frame "UI: Front Panel State" {
        # "Argument"
        # "Set Front Panel Open or Closed\n(Usage: \"UI: Front Panel State >> Open|Close\")"
        n194 = Unbundle By Name(w443) -> ("Core.Current VI Reference"=w442:refnum<vi>)
        n195 = case shown="\"Open\", \"Standard\", Default" w441 {
          tunnel: w445 -> [w452 w466 w478 w491 w504]
          tunnel: [w453 w467 w479 w492 w505] -> w444
          tunnel: w442 -> [w450 w464 w476 w489 w502]
          frame "Open", "Standard", Default {
            w446 = T4."Standard" ("State")
            n196 = property class="VI"(reference=w450, error in=w452) -> (reference out=w449:refnum<vi>, error out=w451:errorcluster, "FP.State"=w448:T4)
            n197 = Not Equal?(x=w448, y=w446) -> (x != y?=w447:bool)
            n198 = case shown="True" w447 {
              tunnel: [w458 w459] -> w453
              tunnel: w451 -> [w457 w459]
              tunnel: w449 -> [w455 _]
              tunnel: w446 -> [w454 _]
              frame True {
                n199 = invoke class="VI" method="FP.Open"(reference=w455, error in=w457, "Activate"=TRUE, "State"=w454) -> (error out=w458:errorcluster)  [unwired: 1 in, 4 out]
              }
              frame False {
              }
            }
          }
          frame "Close", "Closed" {
            n200 = property class="VI"(reference=w464, error in=w466) -> (reference out=w463:refnum<vi>, error out=w465:errorcluster, "FP.State"=w461:T4)
            n201 = Not Equal?(x=w461, y=T4."Closed" ("Front Panel Window:State")) -> (x != y?=w460:bool)
            n202 = case shown="True" w460 {
              tunnel: [w468 w471] -> w467
              tunnel: w465 -> [w468 w470]
              tunnel: w463 -> [_ w469]
              frame False {
              }
              frame True {
                n203 = invoke class="VI" method="FP.Close"(reference=w469, error in=w470) -> (error out=w471:errorcluster)  [unwired: 1 in, 2 out]
              }
            }
          }
          frame "Hidden", "Hide" {
            w472 = T4."Hidden" ("State")
            n204 = property class="VI"(reference=w476, error in=w478) -> (reference out=w475:refnum<vi>, error out=w477:errorcluster, "FP.State"=w474:T4)
            n205 = Not Equal?(x=w474, y=w472) -> (x != y?=w473:bool)
            n206 = case shown="True" w473 {
              tunnel: [w483 w484] -> w479
              tunnel: w477 -> [w482 w484]
              tunnel: w475 -> [w481 _]
              tunnel: w472 -> [w480 _]
              frame True {
                n207 = invoke class="VI" method="FP.Open"(reference=w481, error in=w482, "State"=w480) -> (error out=w483:errorcluster)  [unwired: 2 in, 4 out]
              }
              frame False {
              }
            }
          }
          frame "Minimize", "Minimized" {
            w485 = T4."Minimized" ("State")
            n208 = property class="VI"(reference=w489, error in=w491) -> (reference out=w488:refnum<vi>, error out=w490:errorcluster, "FP.State"=w487:T4)
            n209 = Not Equal?(x=w487, y=w485) -> (x != y?=w486:bool)
            n210 = case shown="True" w486 {
              tunnel: [w496 w497] -> w492
              tunnel: w490 -> [w495 w497]
              tunnel: w488 -> [w494 _]
              tunnel: w485 -> [w493 _]
              frame True {
                n211 = invoke class="VI" method="FP.Open"(reference=w494, error in=w495, "State"=w493) -> (error out=w496:errorcluster)  [unwired: 2 in, 4 out]
              }
              frame False {
              }
            }
          }
          frame "Maximize", "Maximized" {
            w498 = T4."Maximized" ("State")
            n212 = property class="VI"(reference=w502, error in=w504) -> (reference out=w501:refnum<vi>, error out=w503:errorcluster, "FP.State"=w500:T4)
            n213 = Not Equal?(x=w500, y=w498) -> (x != y?=w499:bool)
            n214 = case shown="True" w499 {
              tunnel: [w509 w510] -> w505
              tunnel: w503 -> [w508 w510]
              tunnel: w501 -> [w507 _]
              tunnel: w498 -> [w506 _]
              frame True {
                n215 = invoke class="VI" method="FP.Open"(reference=w507, error in=w508, "State"=w506) -> (error out=w509:errorcluster)  [unwired: 2 in, 4 out]
              }
              frame False {
              }
            }
          }
        }
        n216 = call "Enqueue Multiple States.vi"("queue in"=w440) -> ()  [unwired: 14 in, 1 out]
      }
      frame "UI: Interlocks" {
        n217 = Unbundle By Name(w518) -> ("Active Resource.type"=w512:u32, "Path"=w515:path)
        n218 = call <vilib>:"Check if File or Folder Exists.vi"("error in (no error)"=w522, "path"=w515) -> ("error out"=w516:errorcluster, "file or folder exists?"=w514:bool)  [unwired: 7 in, 1 out]
        n219 = call-poly <userlib>:"MGI Gray if.vi"("Boolean"=w514) -> ("Disabled"=w513:T8)
        n220 = Type Cast(x=w512) -> (*(type *) &x=w521:string)  [unwired: 1 in]
        n221 = Greater Than 0?(x=w512) -> (x > 0?=w511:bool)
        n222 = Search 1D Array(1D array=string[] ["BDHX", "BDHT", "FPHX", "FPHT"], element=w521) -> (index of element=w520:i32)  [unwired: 1 in]
        n223 = Greater Or Equal To 0?(x=w520) -> ()  [unwired: 1 out]
        n224 = call-poly <userlib>:"MGI Gray if.vi"("Boolean"=w511) -> ("Disabled"=w517:T8)
        n225 = property on="Load" class="Bool"("DisabledEnum"=w513) -> ()  [unwired: 2 in, 2 out]
        n226 = property on="Copy" class="Bool"("DisabledEnum"=w517) -> ()  [unwired: 2 in, 2 out]
        n227 = property on="Paste" class="Bool"("DisabledEnum"=w517) -> ()  [unwired: 2 in, 2 out]
      }
      frame "UI: Display Resource" {
        n228 = Unbundle By Name(w523) -> ("Active Resource.binary data"=w524:string, "Active Resource.type"=w525:u32, "Active Resource.id"=w526:i32, "Active Resource.name"=w527:string)
        n229 = local write "ID"(w526) -> ()
        n230 = local write "Name"(w527) -> ()
        n231 = Type Cast(x=w525) -> (*(type *) &x=w528:string)  [unwired: 1 in]
        n232 = local write "Data"(w524) -> ()
        n233 = local write "Type"(w528) -> ()
      }
      frame "UI: Confirm Save" {
        n234 = Unbundle By Name(w535) -> ("All Resources"=w533:T1[], "Path"=w534:path)
        n235 = call <vilib>:"Check if File or Folder Exists.vi"("error in (no error)"=w532, "path"=w534) -> ("error out"=w531:errorcluster, "file or folder exists?"=w536:bool, "dup path"=w538:path)  [unwired: 7 in]
        n236 = case shown="True" w536 {
          tunnel: [TRUE ("T button?") w547] -> w537
          frame False {
          }
          frame True {
            n237 = Two Button Dialog(message="This file already exists. Overwrite it?", 1:"No", 2:"Yes" ("T button name (\"OK\")")) -> (T button?=w547:bool)
          }
        }
        n238 = case shown="True" w537 {
          tunnel: w538 -> [_ w543]
          tunnel: w533 -> [_ w542]
          tunnel: w531 -> [w539 w541]
          tunnel: [w539 w540] -> w530
          frame False {
          }
          frame True {
            n239 = call "Save Resource File.vi"("error in (no error)"=w541, "Path"=w543, "File type"="File type", "Resources"=w542) -> ("error out"=w540:errorcluster)  [unwired: 7 in]
          }
        }
      }
      frame "UI: Confirm Fix" {
        n240 = in-place {
          # "cancel?"
          n241 = in-place-cluster #12(w551) -> ("All Resources"=w555:T1[], "File Type"=w554:string)
          n242 = call-poly <vilib>:"Three Button Dialog.vi"("message"="Have you modified LIBN and/or LVSR at all?") -> ("Which Button?"=w560:T7)  [unwired: 10 in]
          n243 = case shown="\"Left Button\"" w560 {
            tunnel: [w568 FALSE ("Canceled?") TRUE ("Canceled?")] -> w559
            tunnel: [w567 _ _] -> w561
            tunnel: w555 -> [w564 _ _]
            tunnel: [w563 _ _] -> w558
            tunnel: w554 -> [w562 _ _]
            frame "Left Button" {
              # "<--"
              n244 = call <vilib>:"Generate Temporary File Path.vi"("Temporary File Extension (tmp)"="vi") -> ("Unique Temporary File Path"=w566:path)  [unwired: 9 in, 1 out]
              n245 = stacked-sequence {
                seq-local: [w570 _] -> [_ w573]
                tunnel: w566 -> [w572 w575]
                tunnel: w564 -> [w571 _]
                tunnel: [_ w576] -> w563
                tunnel: w562 -> [w569 _]
                frame #0 {
                  n246 = call "Save Resource File.vi"("Path"=w572, "File type"=w569, "Resources"=w571) -> ("error out"=w570:errorcluster)  [unwired: 8 in]
                }
                frame #1 {
                  n247 = Open VI Reference(vi path=w575, error in (no error)=w573) -> (vi reference=w576:refnum<vi>, error out=w574:errorcluster)  [unwired: 4 in]
                  n248 = call <vilib>:"Clear Errors.vi"("error in (no error)"=w574) -> ()  [unwired: 5 in, 2 out]
                }
              }
              n249 = call "Prompt for Terminal Counts.vi"("Reference VI"=w563) -> ("Canceled?"=w568:bool, "Terminal Counts"=w567:T9)  [unwired: 9 in]
            }
            frame "Center Button" {
            }
            frame "Right Button", "Window Close" {
            }
          }
          n250 = Close Reference(reference=w558) -> (error out=w557:errorcluster)  [unwired: 1 in]
          n251 = call <vilib>:"Clear Errors.vi"("error in (no error)"=w557) -> ()  [unwired: 5 in, 2 out]
          n252 = case shown="False" w559 {
            tunnel: w555 -> [w584 w585]
            tunnel: [w583 w585] -> w553
            tunnel: w561 -> [w582 _]
            tunnel: w560 -> [w580 _]
            frame False {
              n253 = Equal?(x=w580, y=T7."Center Button" ("Which Button?")) -> (x = y?=w579:bool)
              n254 = call "Fix BDPW Checksum.vi"("Terminal Counts"=w582, "Only fix 3rd hash (F)"=w579, "Resources"=w584) -> ("Resources out"=w583:T1[])  [unwired: 7 in, 1 out]
            }
            frame True {
            }
          }
          n255 = in-place-cluster #12("All Resources"=w553, "File Type"=w554) -> (w550:T2)
        }
      }
      frame "---------- Macro ----------" {
        # "Do not put any code in this frame.\n(It is a separator no-op. You can make a copy of this frame to create a new Macro frame)"
        n256 = call "Enqueue Multiple States.vi"("queue in"=w586) -> ()  [unwired: 14 in, 1 out]
      }
      frame "Macro: Initialize" {
        w591 = "Data: Initialize\nInitialize Core Data\nUI: Initialize\nUI: Front Panel State >> Open\n%s\nUI: Interlocks"  # Data: Initialize Initialize Core Data UI: Initialize UI: Front Panel State >> Open %s UI: Interlocks
        # "Initialization Macro\n(This is called once, when the VI starts)"
        n257 = Select(t="Data: Load from Path", s="Load from Initial Path (F)", f="Data: Refresh Resources") -> (s? t:f=w590:string)
        n258 = Format Into String(format string=w591, w590) -> (resulting string=w589:string)  [unwired: 2 in, 1 out]
        n259 = call "Enqueue Multiple States.vi"("State(s) at Front"=w589, "queue in"=w595) -> ()  [unwired: 13 in, 1 out]
      }
      frame "Macro: Exit" {
        # "Exit Macro\n(This is called once, when the VI exits)"
        n260 = Unbundle By Name(w606) -> ("Core.Close Panel on Exit?"=w605:bool)
        n261 = property on="Resources" class="MCListbox (strict)"("ItemNames"=string[][] [] ("Item Names")) -> ()  [unwired: 2 in, 2 out]
        n262 = Select(t="UI: Front Panel State >> Close\n", s=w605, f="") -> (s? t:f=w601:string)
        n263 = Concatenate Strings(w601, "Data: Cleanup\nExit") -> (w599:string)
        n264 = call "Enqueue Multiple States.vi"("State(s) at Front"=w599, "queue in"=w602) -> ()  [unwired: 13 in, 1 out]
      }
    }
  }
  n265 = Merge Errors(w12, w13) -> (w11:errorcluster)
  n266 = Release Queue(queue=w10, error in (no error)=w11) -> (error out=w5:errorcluster)  [unwired: 1 in, 2 out]
  n267 = Unregister For Events(event registration refnum=w4, error in=w5) -> ()  [unwired: 1 out]
  n268 = Unbundle By Name(w2) -> ("All Resources"=→"Final Resources":T1[])
